vi "Periodic Tasks.vi"(8 "error in":errorcluster) -> ()   [LabVIEW 2014]
doc: "This VI runs in parallel to other tasks. It can contain as many user-defined periodic loops as you need. These can carry out PID or other sorts of timed response."
uses:
  <vilib>/Rock Robotics/WPI/Compressor/WPI_CompressorGetSetRefNum.vi
  <vilib>/Rock Robotics/Network Tables/SD Write Boolean.vi
  Global Variables.vi
  <vilib>/Rock Robotics/Network Tables/SD Write Number.vi
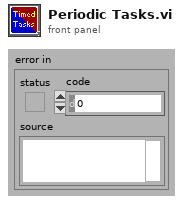
[diagram p1: front panel]
types:
  T1 = typedef "WPI_EncoderDevRef.ctl" = cluster{"DevStatus":errorcluster, "EncoderIndex":T2, "CounterIndex":T3, "DistancePerCount":dbl, "Decoding Type":T4}
  T2 = typedef "FPGA_EncoderIdx.ctl" = enum8{"Enc 0", "Enc 1", "Enc 2", "Enc 3", "Enc 4", "Enc 5", "Enc 6", "Enc 7", "Invalid"}
  T3 = typedef "FPGA_CounterCtrSystemIndex.ctl" = enum8{"Ctr 0", "Ctr 1", "Ctr 2", "Ctr 3", "Ctr 4", "Ctr 5", "Ctr 6", "Ctr 7", "Invalid"}
  T4 = typedef "WPI_EncoderType.ctl" = enum16{"1x", "2x", "4x"}
  T5 = typedef "WPI_CompressorDevRef.ctl" = cluster{"DevStatus":errorcluster, "Pneumatics Control Module":u8}
  T6 = typedef "WPI_GyroDevRef.ctl" = cluster{"DevStatus":errorcluster, "Analog Module":T7, "Analog Channel":T8, "Offset":dbl, "Gain (VoltsPerDegree/Second)":dbl}
  T7 = typedef "FPGA_TypedefAnalogModule.ctl" = enum16{"Controller 1"}
  T8 = typedef "FPGA_AIChannel.ctl" = enum8{"AI 0", "AI 1", "AI 2", "AI 3", "AI MXP 0", "AI MXP 1", "AI MXP 2", "AI MXP 3", "Invalid"}
  T9 = typedef "WPI_DigitalInputDevRef.ctl" = cluster{"DevStatus":errorcluster, "DIO Channel":T10, "Controller":T11}
  T10 = typedef "FPGA_DIOChannel.ctl" = enum8{"DIO 0", "DIO 1", "DIO 2", "DIO 3", "DIO 4", "DIO 5", "DIO 6", "DIO 7", "DIO 8", "DIO 9", "DIO MXP 0", "DIO MXP 1", "DIO MXP 2", "DIO MXP 3", "DIO MXP 4", "DIO MXP 5", "DIO MXP 6", "DIO MXP 7", "DIO MXP 8", "DIO MXP 9", "DIO MXP 10", "DIO MXP 11", "DIO MXP 12", "DIO MXP 13", "DIO MXP 14", "DIO MXP 15", "Invalid"}
  T11 = typedef "FPGA_TypedefDigitalModule.ctl" = enum16{"Controller 1"}
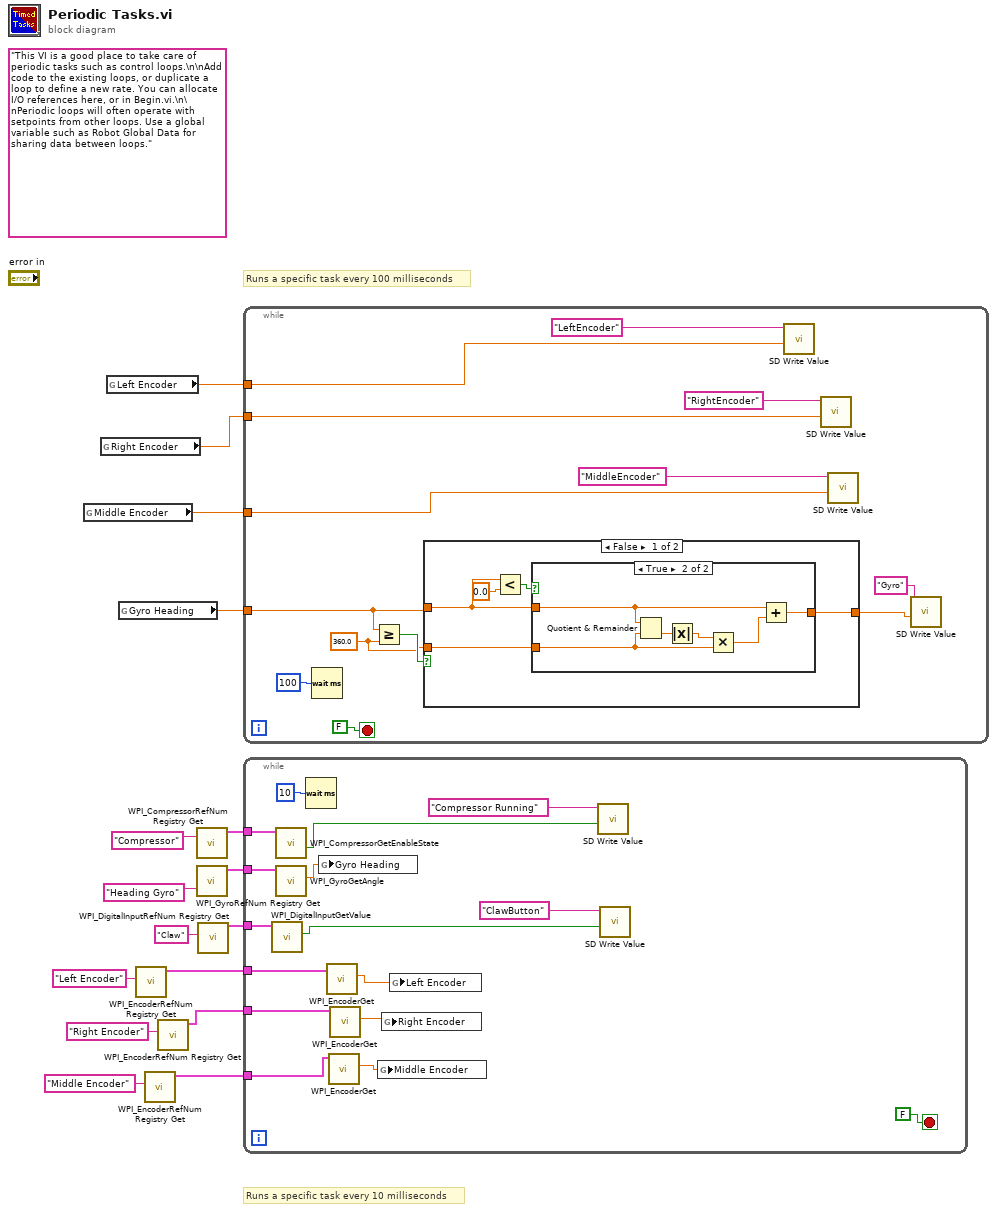
[diagram p0: block diagram]
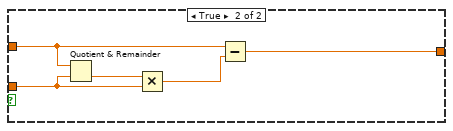
[diagram p3: hidden frame]
diagram:
  (unwired) "This VI is a good place to take care of periodic tasks such as control loops.\n\nAdd code to the existing loops, or duplicate a loop to define a new rate. You can allocate I/O references here, or in Begin.vi.\n\nPeriodic loops will often operate with setpoints from other loops. Use a global variable such as Robot Global Data for sharing data between loops."
  # "Runs a specific task every 100 milliseconds"
  # "Runs a specific task every 10 milliseconds"
  n1 = global read "Global Variables.vi" "Middle Encoder"() -> (w3:dbl)
  n2 = global read "Global Variables.vi" "Right Encoder"() -> (w4:dbl)
  n3 = global read "Global Variables.vi" "Left Encoder"() -> (w5:dbl)
  n4 = global read "Global Variables.vi" "Gyro Heading"() -> (w6:dbl)
  n5 = call <vilib>:"WPI_EncoderRefNum Registry Get.vi"("refnum name"="Left Encoder") -> ("EncoderDevRef"=w9:T1)  [unwired: 9 in, 1 out]
  n6 = call <vilib>:"WPI_EncoderRefNum Registry Get.vi"("refnum name"="Middle Encoder") -> ("EncoderDevRef"=w7:T1)  [unwired: 9 in, 1 out]
  n7 = call <vilib>:"WPI_EncoderRefNum Registry Get.vi"("refnum name"="Right Encoder") -> ("EncoderDevRef"=w8:T1)  [unwired: 9 in, 1 out]
  n8 = call <vilib>:"WPI_CompressorRefNum Registry Get.vi"("refnum name"="Compressor") -> ("CompressorDevRef"=w13:T5)  [unwired: 9 in, 1 out]
  n9 = call <vilib>:"WPI_GyroRefNum Registry Get.vi"("refnum name"="Heading Gyro") -> ("GyroDevRef"=w15:T6)  [unwired: 9 in, 1 out]
  n10 = call <vilib>:"WPI_DigitalInputRefNum Registry Get.vi"("refnum name"="Claw") -> ("DigitalInputDevRef"=w1:T9)  [unwired: 9 in, 1 out]
  n11 = while {
    tunnel: w6 -> [w25]
    tunnel: w5 -> [w21]
    tunnel: w4 -> [w20]
    tunnel: w3 -> [w19]
    stop <- FALSE stop-if-true
    w26 = 360.0 ("y")
    n12 = Wait (ms)(milliseconds to wait=u32 100) -> ()  [unwired: 1 out]
    n13 = Greater Or Equal?(x=w25, y=w26) -> (x >= y?=w27:bool)
    n14 = case shown="False" w27 {
      tunnel: w25 -> [w32 w44]
      tunnel: w26 -> [w31 w45]
      tunnel: [w30 w42] -> w18
      frame False {
        n15 = Less?(x=w32, y=0.0) -> (x < y?=w34:bool)
        n16 = case shown="True" w34 {
          tunnel: w32 -> [w35 w41]
          tunnel: w31 -> [_ w38]
          tunnel: [w35 w40] -> w30
          frame False {
          }
          frame True {
            n17 = Quotient & Remainder(x=w41, y=w38) -> (floor(x/y)=w37:dbl)  [unwired: 1 out]
            n18 = Absolute Value(x=w37) -> (abs(x)=w36:dbl)
            n19 = Multiply(x=w36, y=w38) -> (x*y=w39:dbl)
            n20 = Add(x=w41, y=w39) -> (x+y=w40:dbl)
          }
        }
      }
      frame True {
        n21 = Quotient & Remainder(x=w44, y=w45) -> (floor(x/y)=w46:dbl)  [unwired: 1 out]
        n22 = Multiply(x=w46, y=w45) -> (x*y=w43:dbl)
        n23 = Subtract(x=w44, y=w43) -> (x-y=w42:dbl)
      }
    }
    n24 = call-poly <vilib>:"SD Write Value.vi"("Numeric"=w21, "Name"="LeftEncoder" ("refnum name")) -> ()  [unwired: 8 in, 2 out]
    n25 = call-poly <vilib>:"SD Write Value.vi"("Numeric"=w20, "Name"="RightEncoder" ("refnum name")) -> ()  [unwired: 8 in, 2 out]
    n26 = call-poly <vilib>:"SD Write Value.vi"("Numeric"=w19, "Name"="MiddleEncoder" ("refnum name")) -> ()  [unwired: 8 in, 2 out]
    n27 = call-poly <vilib>:"SD Write Value.vi"("Numeric"=w18, "Name"="Gyro") -> ()  [unwired: 8 in, 2 out]
  }
  n28 = while {
    tunnel: w15 -> [w60]
    tunnel: w13 -> [w59]
    tunnel: w9 -> [w58]
    tunnel: w8 -> [w57]
    tunnel: w7 -> [w56]
    tunnel: w1 -> [w47]
    stop <- FALSE stop-if-true
    n29 = call <vilib>:"WPI_DigitalInputGetValue.vi"("DigitalInputDevRef"=w47) -> ("Value"=w48:bool)  [unwired: 8 in, 2 out]
    n30 = call <vilib>:"WPI_CompressorGetEnableState.vi"("CompressorDevRef"=w59) -> ("Compressor Running"=w52:bool)  [unwired: 7 in, 3 out]
    n31 = call <vilib>:"WPI_GyroGetAngle.vi"("GyroDevRef"=w60) -> ("Angle"=w51:dbl)  [unwired: 7 in, 3 out]
    n32 = Wait (ms)(milliseconds to wait=u32 10) -> ()  [unwired: 1 out]
    n33 = global write "Global Variables.vi" "Gyro Heading"(w51) -> ()
    n34 = call <vilib>:"WPI_EncoderGet.vi"("EncoderDevRef"=w58) -> ("Distance"=w53:dbl)  [unwired: 5 in, 5 out]
    n35 = call <vilib>:"WPI_EncoderGet.vi"("EncoderDevRef"=w56) -> ("Distance"=w55:dbl)  [unwired: 5 in, 5 out]
    n36 = call <vilib>:"WPI_EncoderGet.vi"("EncoderDevRef"=w57) -> ("Distance"=w54:dbl)  [unwired: 5 in, 5 out]
    n37 = global write "Global Variables.vi" "Middle Encoder"(w55) -> ()
    n38 = global write "Global Variables.vi" "Right Encoder"(w54) -> ()
    n39 = global write "Global Variables.vi" "Left Encoder"(w53) -> ()
    n40 = call-poly <vilib>:"SD Write Value.vi"("Boolean"=w52, "Name"="Compressor Running") -> ()  [unwired: 8 in, 2 out]
    n41 = call-poly <vilib>:"SD Write Value.vi"("Boolean"=w48, "Name"="ClawButton") -> ()  [unwired: 8 in, 2 out]
  }
